vi "WavegenSwitch.vi"(8 "error in (no error)":errorcluster caption="错误输入（无错误）", 9 "output":bool=TRUE, 10 "ch":i32, 11 "ftHandle":u64) -> (0 "error out":errorcluster caption="错误输出", 2 "function out":i32, 3 "ftHandle out":u64)   [LabVIEW 2018]
doc: "Set Wavegen Simple mode configration and output\n0:CH1;1:CH2;2:Both CH1 and CH2"
uses:
  InstrumentsPlayground.lvlib
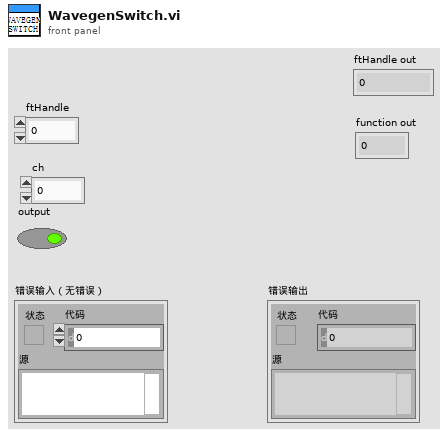
[diagram p1: front panel]
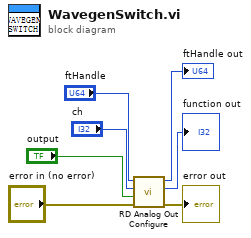
[diagram p0: block diagram]
diagram:
  n1 = call "RD Analog Out Configure.vi"("error in (no error)"="error in (no error)", "output"="output", "ch"="ch", "handle"="ftHandle") -> ("error out"=→"error out":errorcluster, "function return"=→"function out":i32, "handle out"=→"ftHandle out":u64)  [unwired: 5 in]
